vi "Get Command FIFO.vi"(11 "Interface in":refnum<class "Interface.lvclass">) -> (2 "command fifo":refnum<k33>, 3 "Interface out":refnum<class "Interface.lvclass">)   [LabVIEW 2021, in "DSF Core.lvlib" / "Interface.lvclass"]
uses:
  Interface.lvclass
  Interface.lvclass/Interface.ctl
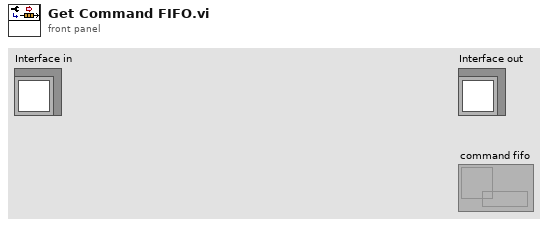
[diagram p1: front panel]
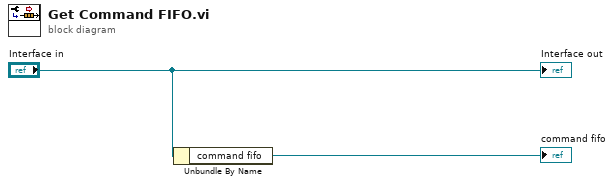
[diagram p0: block diagram]
diagram:
  n1 = Unbundle By Name("Interface in") -> ("command fifo"=→"command fifo":refnum<k33>)
  "Interface out" <- "Interface in"
